vi "mkResetCamera.vi"(11 "IMAQ Refnum in":refnum<k11>) -> (3 "IMAQ Refnum out":refnum<k11>)   [LabVIEW 2011]
panel:
  out "String Read":string
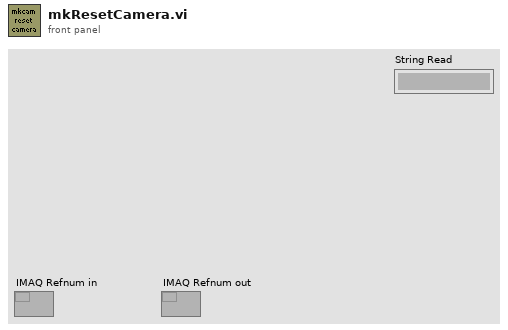
[diagram p1: front panel]
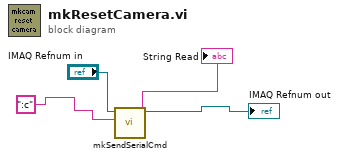
[diagram p0: block diagram]
diagram:
  n1 = call "mkSendSerialCmd.vi"("String"=":c" ("format string"), "IMAQ Refnum in"="IMAQ Refnum in") -> ("String Read"=→"String Read":string, "IMAQ Refnum out"=→"IMAQ Refnum out":refnum<k11>)  [unwired: 6 in, 2 out]
